vi "Check If VIs are Running.vi"(8 "error in (no error)":errorcluster, 10 "State":T1(ring)=enum."Hidden", 11 "Path":path) -> (0 "error out":errorcluster)   [LabVIEW 2015]
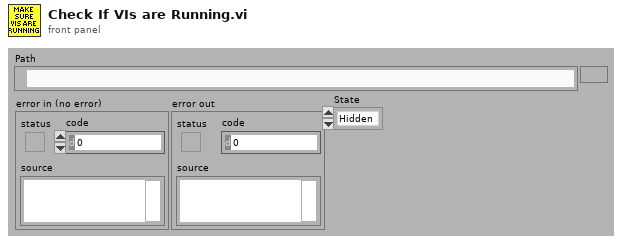
[diagram p1: front panel]
types:
  T1 = enum32{"Invalid", "Standard", "Closed", "Hidden", "Minimized", "Maximized"}
  T2 = enum32{"Bad", "Idle", "Run top level", "Running"}
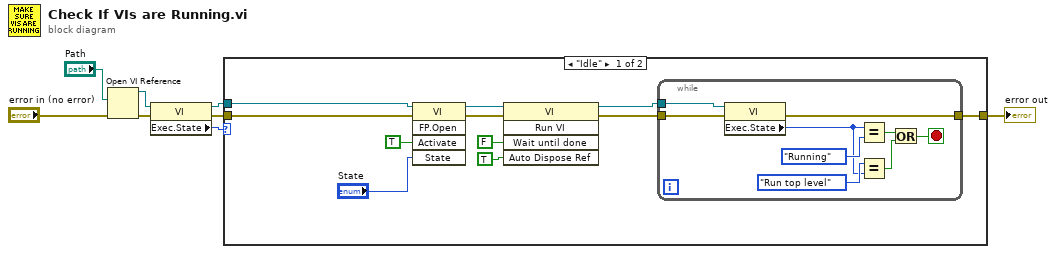
[diagram p0: block diagram]
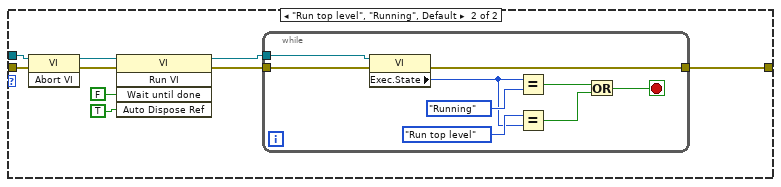
[diagram p2: hidden frame]
diagram:
  n1 = Open VI Reference(vi path="Path", error in (no error)="error in (no error)") -> (vi reference=w7:refnum<vi>, error out=w6:errorcluster)  [unwired: 4 in]
  n2 = property class="VI"(reference=w7, error in=w6) -> (reference out=w3:refnum<vi>, error out=w2:errorcluster, "Exec.State"=w5:T2)
  n3 = case shown="\"Idle\"" w5 {
    tunnel: w3 -> [w19 w32]
    tunnel: w2 -> [w18 w30]
    tunnel: [w9 w33] -> w1
    frame "Idle" {
      n4 = invoke class="VI" method="FP.Open"(reference=w19, error in=w18, "Activate"=TRUE ("Activate?"), "State"="State") -> (reference out=w15:refnum<vi>, error out=w14:errorcluster)  [unwired: 1 in, 3 out]
      n5 = invoke class="VI" method="Run VI"(reference=w15, error in=w14, "Wait until done"=FALSE ("Wait Until Done"), "Auto Dispose Ref"=TRUE ("Auto Dispose Reference")) -> (reference out=w11:refnum<vi>, error out=w10:errorcluster)  [unwired: 1 in, 3 out]
      n6 = while {
        tunnel: w11 -> [w28]
        tunnel: w10 -> [w27]
        tunnel: [w26] -> w9
        stop <- w20 stop-if-true
        n7 = property class="VI"(reference=w28, error in=w27) -> (error out=w26:errorcluster, "Exec.State"=w23:T2)  [unwired: 1 out]
        n8 = Equal?(x=w23, y=T2."Running" ("Execution:State")) -> (x = y?=w21:bool)
        n9 = Equal?(x=T2."Run top level" ("Execution:State"), y=w23) -> (x = y?=w22:bool)
        n10 = Or(x=w21, y=w22) -> (x .or. y?=w20:bool)
      }
    }
    frame "Run top level", "Running", Default {
      n11 = invoke class="VI" method="Abort VI"(reference=w32, error in=w30) -> (reference out=w31:refnum<vi>, error out=w29:errorcluster)  [unwired: 1 in, 1 out]
      n12 = invoke class="VI" method="Run VI"(reference=w31, error in=w29, "Wait until done"=FALSE ("Wait Until Done"), "Auto Dispose Ref"=TRUE ("Auto Dispose Reference")) -> (reference out=w35:refnum<vi>, error out=w34:errorcluster)  [unwired: 1 in, 3 out]
      n13 = while {
        tunnel: w35 -> [w46]
        tunnel: w34 -> [w45]
        tunnel: [w44] -> w33
        stop <- w38 stop-if-true
        n14 = property class="VI"(reference=w46, error in=w45) -> (error out=w44:errorcluster, "Exec.State"=w41:T2)  [unwired: 1 out]
        n15 = Equal?(x=w41, y=T2."Running" ("Execution:State")) -> (x = y?=w39:bool)
        n16 = Equal?(x=T2."Run top level" ("Execution:State"), y=w41) -> (x = y?=w40:bool)
        n17 = Or(x=w39, y=w40) -> (x .or. y?=w38:bool)
      }
    }
  }
  "error out" <- w1
